vi "licdf counter read.vi"(8 "error in (no error)":errorcluster, 9 "out_value":i32, 10 "counter_id":i32, 11 "handle":i32) -> (0 "error out":errorcluster, 1 "out_value out":i32, 3 "function return":i32)   [LabVIEW 2026, in "keynub_licdongle.lvlib"]
doc: "int32_t licdf_counter_read(int32_t handle, int32_t counter_id, int32_t *out_value);"
uses:
  keynub_licdongle.lvlib
  natives/win-x64/keynub_licdongle_flat.dll
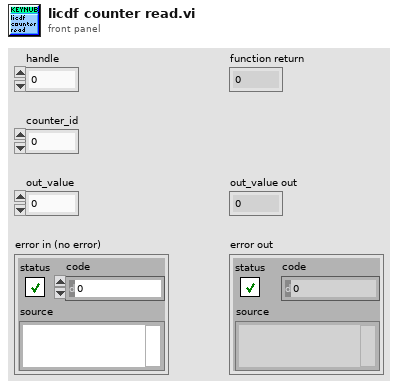
[diagram p1: front panel]
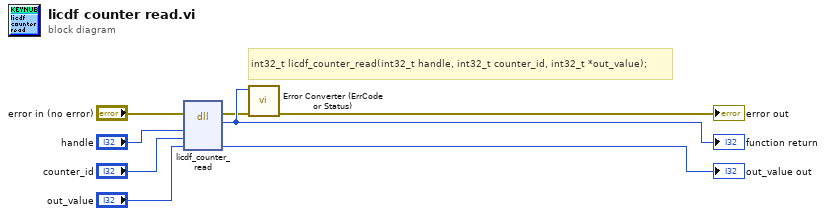
[diagram p0: block diagram]
diagram:
  # "int32_t licdf_counter_read(int32_t handle, int32_t counter_id, int32_t *out_value);"
  n1 = dll-call lib="C:/Austausch/KeyNub/LicenseDongle-PublicSDK/natives/win-x64/keynub_licdongle_flat.*" fn="licdf_counter_read"(error in="error in (no error)", "handle"="handle", "counter_id"="counter_id", "out_value"="out_value") -> (error out=w2:errorcluster, w8:i32, "out_value"=→"out_value out":i32)  [unwired: 4 in, 1 out]
  "function return" <- w8
  n2 = call "Error Converter (ErrCode or Status).vi"("error in (no error)"=w2, "error code"=w8) -> ("error out"=→"error out":errorcluster)  [unwired: 9 in]
